vi "Digitizer Channel UI.vi"() -> ()   [LabVIEW 2025, in "Digitizer.lvlib" / "Digitizer Channel.lvclass"]
doc: "Copyright 2017 National Instruments Corporation\n\nLicensed under the Apache License, Version 2.0 (the \"License\"); you may not use this file except in compliance with the License. You may obtain a copy of the License at http://www.apache.org/licenses/LICENSE-2.0\nUnless required by applicable law or agreed to in writing, software distributed under the License is distributed on an \"AS IS\" BASIS, WITHOUT WARRANTIES OR CONDITIONS OF ANY KIND, either express or implied. See the License for the specific language governing permissions and limitations under the License."
uses:
  Digitizer Channel.lvclass
  Users/Public/Documents/Sandia National Labs/TSS Plugin/CEF.lvlibp/Node/NodeRef.ctl
  Users/Public/Documents/Sandia National Labs/TSS Plugin/CEF.lvlibp/Node/CEF_Node.lvclass
  Users/Public/Documents/Sandia National Labs/TSS Plugin/CEF.lvlibp/Node/mainQref.ctl
  Users/Public/Documents/Sandia National Labs/TSS Plugin/CEF.lvlibp/Node/UserEventRef.ctl
  Users/Public/Documents/Sandia National Labs/TSS Plugin/Abstract Engine.lvlibp/Plugin/Abstract/Channel configuration/Default Channel.ctl
  Digitizer Channel configuration/Digitizer Channel Setting.ctl
  Digitizer Channel.lvclass/Digitizer Channel.ctl
  Digitizer Channel configuration/Digitizer Channel configuration.lvclass/Digitizer Channel configuration.ctl
  Digitizer Channel configuration/Read Digitizer Channel.vi
  Digitizer Channel configuration/Write Digitizer Channel.vi
  <vilib>/Utility/error.llb/Trim Whitespace One-Sided.vi
  Digitizer Channel configuration/Digitizer Channel configuration.lvclass
  Users/Public/Documents/Sandia National Labs/TSS Plugin/Abstract Engine.lvlibp/Plugin/Abstract/Channel configuration/Read Channel Setting.vi
  Users/Public/Documents/Sandia National Labs/TSS Plugin/Abstract Engine.lvlibp/Plugin/Abstract/Channel configuration/Write Channel Setting.vi
  Users/Public/Documents/Sandia National Labs/TSS Plugin/Abstract Engine.lvlibp/Plugin/Abstract/Channel configuration/Channel configuration.lvclass
panel:
  in  "Digitizer Channel":cluster{"Default":T1, "Setting":T2}={"Default"={"Address"="None", "SW Alias"="None", "Enabled"=TRUE, "Type"="None", "Description"="* Type = Channel Class"}, "Setting"={"Max"=0.0, "Min"=0.0, "Data Reduction"="Average", "Averging Points"=1000, "Decimate Interval"=0, "Aperture Options"={"Tolerance"=0, "Burst"=0, "Min SampleRate"=0, "Min SampleIndex"=0}}} {"Setting"."Decimate Interval" format="%.0p"; "Setting"."Averging Points" format="%.0p"; "Setting"."Aperture Options"."Min SampleIndex" format="%.0p"; "Setting"."Aperture Options"."Min SampleRate" format="%.0p"}
  in  "user event":T3
  in  "main queue":T4
  in  "node ref":T5
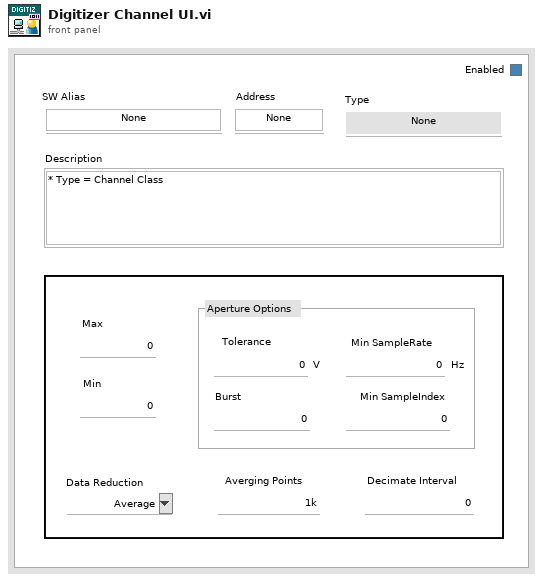
[diagram p1: front panel]
types:
  T1 = typedef "Abstract Engine.lvlibp/Channel configuration.lvclass/Default Channel.ctl" = cluster{"Address":string, "SW Alias":string, "Enabled":bool, "Type":string, "Description":string}
  T2 = typedef "Digitizer.lvlib/Digitizer Channel configuration.lvclass/Digitizer Channel Setting.ctl" = cluster{"Max":dbl, "Min":dbl, "Data Reduction":string, "Averging Points":u32, "Decimate Interval":u32, "Aperture Options":cluster{"Tolerance":u32, "Burst":u32, "Min SampleRate":u32, "Min SampleIndex":u32}}
  T3 = typedef "CEF.lvlibp/CEF_Node.lvclass/UserEventRef.ctl" = refnum<user-event>
  T4 = typedef "CEF.lvlibp/CEF_Node.lvclass/mainQref.ctl" = refnum<queue>
  T5 = typedef "CEF.lvlibp/CEF_Node.lvclass/NodeRef.ctl" = refnum<data-value>
  T6 = cluster{"Channel Setting":T1, "Digitizer Channel":T2}
  T7 = enum8{"Enabled", "Disabled", "Disabled and Grayed Out"}
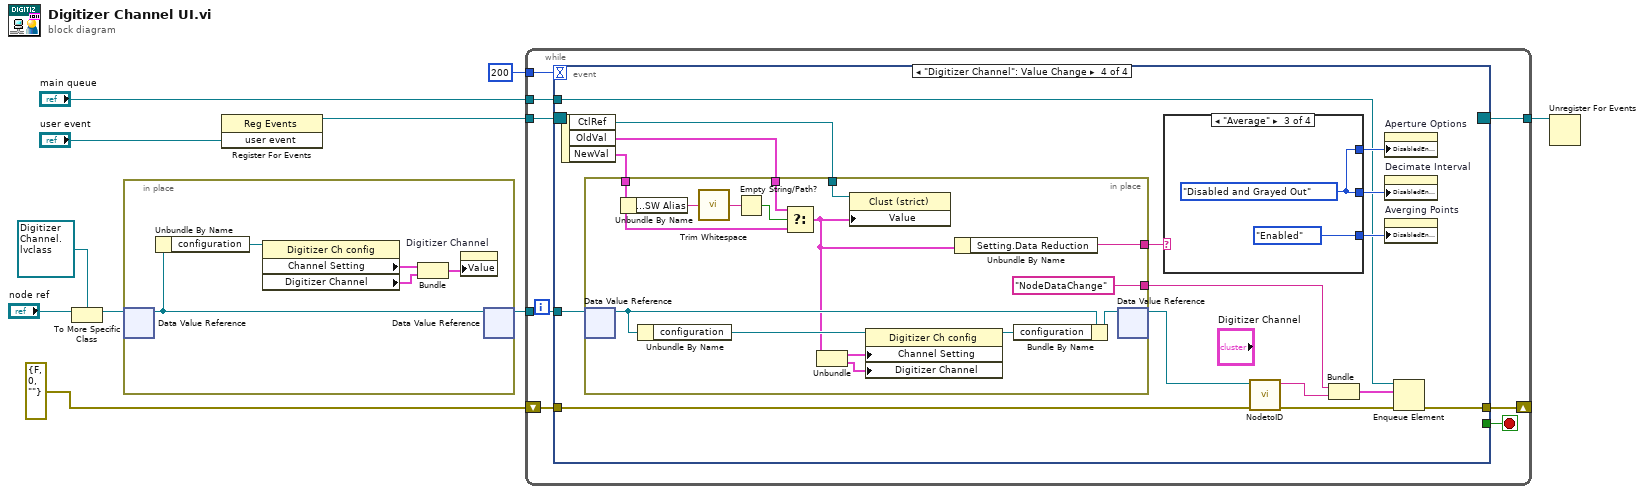
[diagram p0: block diagram]
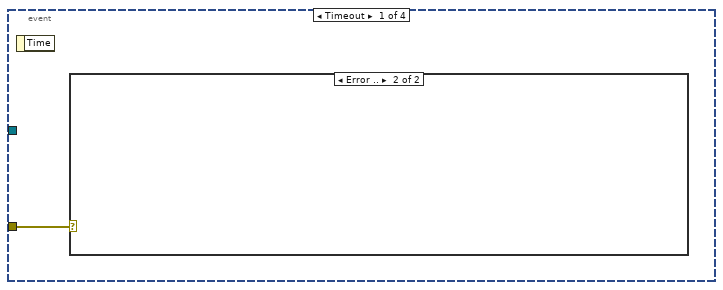
[diagram p2: hidden frame]
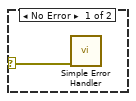
[diagram p3: hidden frame]
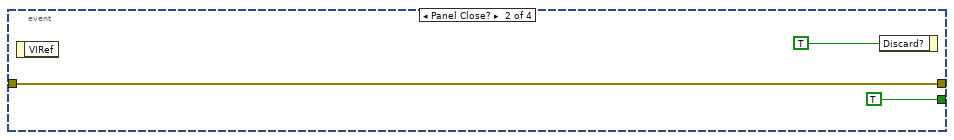
[diagram p4: hidden frame]
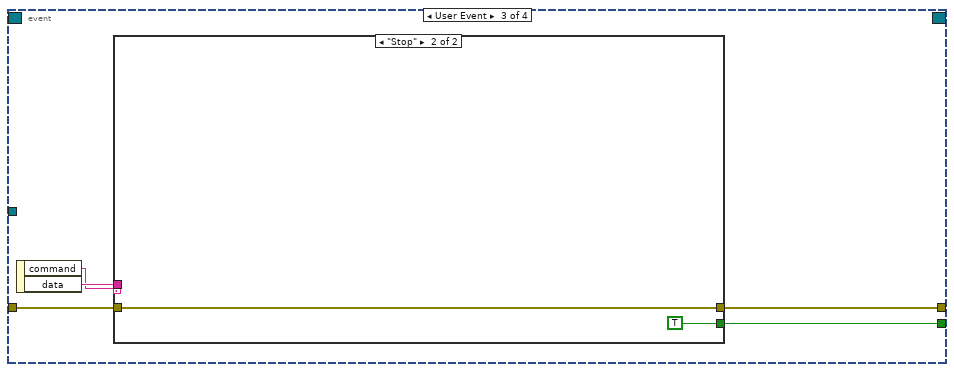
[diagram p5: hidden frame]
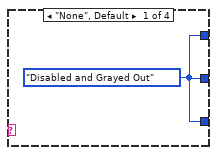
[diagram p7: hidden frame]
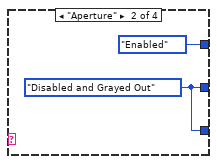
[diagram p8: hidden frame]
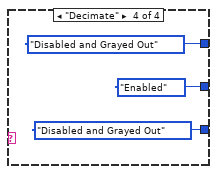
[diagram p9: hidden frame]
diagram:
  n1 = To More Specific Class(target class=refnum<data-value> refnum ("data value reference"), reference="node ref") -> (specific class reference=w5:refnum<data-value>)  [unwired: 1 in, 1 out]
  n2 = in-place {
    # "Initialize the front panel controls when loaded"
    n3 = in-place-dvr #1(w5) -> (w12:refnum<class "Digitizer Channel.lvclass">)  [unwired: 1 out]
    n4 = Unbundle By Name(w12) -> ("configuration"=w15:refnum<class "Digitizer Channel configuration.lvclass">)
    n5 = property class="Digitizer Ch config"(reference=w15) -> ("Channel Setting"=w13:T1, "Digitizer Channel"=w14:T2)  [unwired: 1 in, 2 out]
    n6 = Bundle("Channel Setting"=w13, "Digitizer Channel"=w14) -> (w11:T6)  [unwired: 1 in]
    n7 = property on="Digitizer Channel" class="Clust (strict)"("Value"=w11) -> ()  [unwired: 2 in, 2 out]
    n8 = in-place-dvr #1(w12) -> (w4:refnum<data-value>)  [unwired: 1 out]
  }
  n9 = register-events("user event") -> (reference out=w9:refnum<event-registration>)  [unwired: 2 in, 1 out]
  n10 = while {
    tunnel: w4 -> [w23]
    tunnel: w9 -> [w22]
    tunnel: [w21] -> w8
    tunnel: "main queue" -> [w17]
    shift-right: [w18] -> _
    shift-left: errorcluster {"status"=FALSE, "code"=0, "source"=""} ("error in (no error)") -> [w19]
    tunnel: 200 -> [w16]
    stop <- w20 stop-if-true
    n11 = event shown="[3] \"Digitizer Channel\": Value Change" {
      selector: w22 -> [_ _ _ _]
      dyn-events: [_ _ _ _] -> w21
      timeout: w16 -> [_ _ _ _]
      tunnel: w23 -> [_ _ _ w48]
      tunnel: [_ TRUE w33 _] -> w20
      tunnel: [_ w26 w29 w52] -> w18
      tunnel: w19 -> [w24 w26 w31 w41]
      tunnel: w17 -> [_ _ _ w42]
      event Timeout {
        n12 = event-data() -> ()  [unwired: 1 in, 1 out]
        n13 = case shown="Error .." w24 {
          selector: w24 -> [w25 _]
          frame No Error {
            n14 = call <vilib>:"Simple Error Handler.vi"("error in (no error)"=w25) -> ()  [unwired: 4 in, 5 out]
          }
          frame Error {
          }
        }
      }
      event Panel Close? {
        n15 = event-data() -> ()  [unwired: 1 in, 1 out]
        n16 = event-data("Discard?"=TRUE) -> ()  [unwired: 1 in, 1 out]
      }
      event User Event {
        n17 = event-data() -> ("command"=w30:string, "data"=w32:string)  [unwired: 1 in]
        n18 = case shown="\"Stop\"" w30 {
          tunnel: [_ TRUE] -> w33
          tunnel: w32 -> [_ _]
          tunnel: w31 -> [w34 w35]
          tunnel: [w34 w35] -> w29
          frame Default {
          }
          frame "Stop" {
          }
        }
      }
      event "Digitizer Channel": Value Change {
        n19 = event-data() -> ("CtlRef"=w43:refnum<vi>, "OldVal"=w44:cluster{"Default":T1, "Setting":T2}, "NewVal"=w45:cluster{"Default":T1, "Setting":T2})  [unwired: 1 in]
        n20 = in-place {
          in-place-border: [w67] -> w49
          in-place-border: w45 -> [w60]
          in-place-border: w44 -> [w63]
          in-place-border: w43 -> [w62]
          in-place-border: ["NodeDataChange" ("Message Name")] -> w37
          n21 = in-place-dvr #2(w48) -> (w66:refnum<class "Digitizer Channel.lvclass">)  [unwired: 1 out]
          n22 = Unbundle By Name(w60) -> ("Default.SW Alias"=w61:string)
          n23 = Unbundle By Name(w66) -> ("configuration"=w57:refnum<class "Digitizer Channel configuration.lvclass">)
          n24 = call <vilib>:"Trim Whitespace.vi"("string"=w61) -> ("trimmed string"=w58:string)  [unwired: 1 in]
          n25 = Empty String/Path?(string/path=w58) -> (empty?=w59:bool)
          n26 = Select(t=w63, s=w59, f=w60) -> (s? t:f=w56:cluster{"Default":T1, "Setting":T2})
          n27 = Unbundle(w56) -> ("Default"=w53:T1, "Setting"=w55:T2)
          n28 = property class="Clust (strict)"(reference=w62, "Value"=w56) -> ()  [unwired: 1 in, 2 out]
          n29 = property class="Digitizer Ch config"(reference=w57, "Channel Setting"=w53, "Digitizer Channel"=w55) -> (reference out=w64:refnum<class "Digitizer Channel configuration.lvclass">)  [unwired: 1 in, 1 out]
          n30 = Unbundle By Name(w56) -> ("Setting.Data Reduction"=w67:string)
          n31 = Bundle By Name(cluster=w66, "configuration"=w64) -> (w65:refnum<class "Digitizer Channel.lvclass">)
          n32 = in-place-dvr #2(w65) -> (w46:refnum<data-value>)  [unwired: 1 out]
        }
        n33 = case shown="\"Average\"" w49 {
          tunnel: [w68 T7."Enabled" ("Disabled") w71 T7."Disabled and Grayed Out" ("Disabled")] -> w50
          tunnel: [w68 w69 w71 T7."Enabled" ("Disabled")] -> w51
          tunnel: [w68 w69 T7."Enabled" ("Disabled") T7."Disabled and Grayed Out" ("Disabled")] -> w47
          frame "None", Default {
            w68 = T7."Disabled and Grayed Out" ("Disabled")
          }
          frame "Aperture" {
            w69 = T7."Disabled and Grayed Out" ("Disabled")
          }
          frame "Average" {
            w71 = T7."Disabled and Grayed Out" ("Disabled")
          }
          frame "Decimate" {
          }
        }
        n34 = call "NodetoID.vi"("error in"=w41, "node ref"=w46) -> ("error out"=w39:errorcluster, "ID"=w40:string)  [unwired: 8 in]
        n35 = Bundle("Message Name"=w37, "ID"=w40) -> (w38:cluster{"Message Name":string, "ID":string})  [unwired: 1 in]
        n36 = property on="Aperture Options" class="Clust (strict)"("DisabledEnum"=w50) -> ()  [unwired: 2 in, 2 out]
        n37 = property on="Decimate Interval" class="DigNum (strict)"("DisabledEnum"=w51) -> ()  [unwired: 2 in, 2 out]
        n38 = property on="Averging Points" class="DigNum (strict)"("DisabledEnum"=w47) -> ()  [unwired: 2 in, 2 out]
        n39 = Enqueue Element(queue=w42, element=w38, error in (no error)=w39) -> (error out=w52:errorcluster)  [unwired: 1 in, 2 out]
      }
    }
  }
  n40 = Unregister For Events(event registration refnum=w8) -> ()  [unwired: 1 in, 1 out]
